vi "Q -- check range -- i -- real - window.vi"(4 "window":dbl=inf, 6 "center":dbl=-inf, 8 "default":dbl=nan, 11 "number":dbl=11.0) -> (0 "selector":T1, 2 "in range?":bool=TRUE, 3 "number in range":dbl)   [LabVIEW 2015]
uses:
  comparison control.ctl
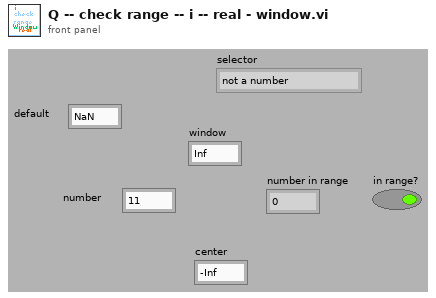
[diagram p1: front panel]
types:
  T1 = typedef "comparison control.ctl" = enum16{"not a number", "above", "in range", "below"}
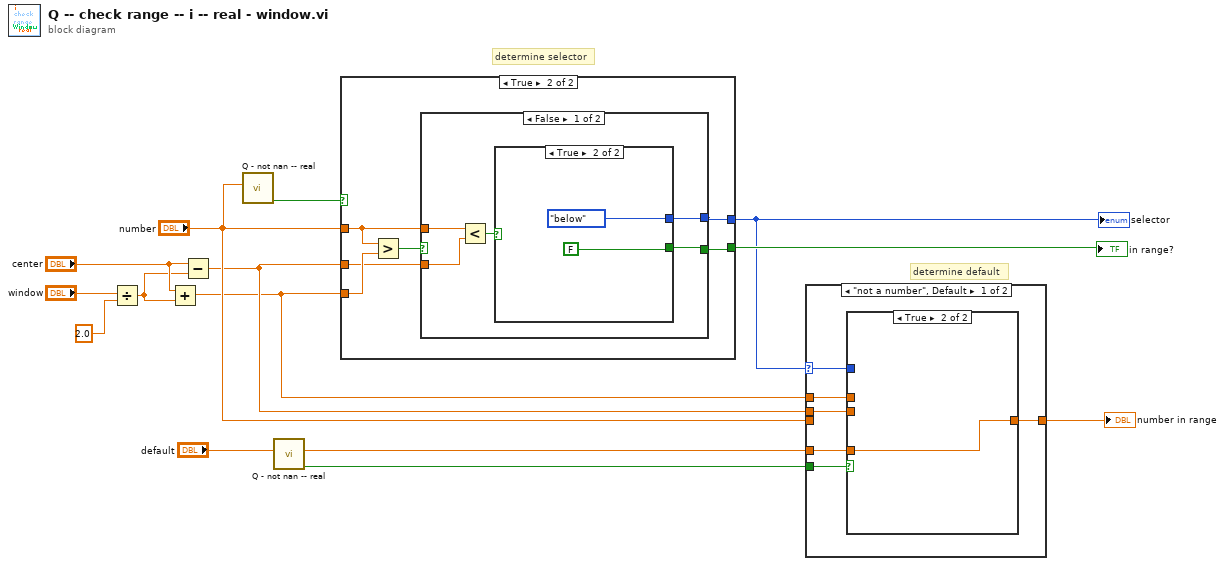
[diagram p0: block diagram]
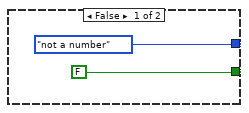
[diagram p5: hidden frame]
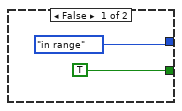
[diagram p6: hidden frame]
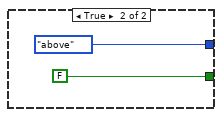
[diagram p7: hidden frame]
diagram:
  # "determine default"
  # "determine selector"
  n1 = Divide(x="window", y=2.0) -> (x/y=w3:dbl)
  n2 = Add(x="center", y=w3) -> (x+y=w1:dbl)
  n3 = Subtract(x="center", y=w3) -> (x-y=w2:dbl)
  n4 = call "Q - not nan -- real.vi"("Numeric"="number") -> ("Boolean"=w12:bool)  [unwired: 9 in, 1 out]
  n5 = call "Q - not nan -- real.vi"("Numeric"="default") -> ("Boolean"=w8:bool, "out"=w7:dbl)  [unwired: 9 in]
  n6 = case shown="True" w12 {
    tunnel: w1 -> [_ w21]
    tunnel: w2 -> [_ w18]
    tunnel: [FALSE w17] -> w14
    tunnel: [comparison_control."not a number" ("selector") w22] -> w11
    tunnel: "number" -> [_ w19]
    frame False {
    }
    frame True {
      n7 = Greater?(x=w19, y=w21) -> (0:w20:bool)
      n8 = case shown="False" w20 {
        tunnel: [w27 comparison_control."above" ("selector")] -> w22
        tunnel: w19 -> [w26 _]
        tunnel: w18 -> [w25 _]
        tunnel: [w23 FALSE] -> w17
        frame False {
          n9 = Less?(x=w26, y=w25) -> (x < y?=w24:bool)
          n10 = case shown="True" w24 {
            tunnel: [comparison_control."in range" ("selector") comparison_control."below" ("selector")] -> w27
            tunnel: [TRUE FALSE] -> w23
            frame False {
            }
            frame True {
            }
          }
        }
        frame True {
        }
      }
    }
  }
  "in range?" <- w14
  "selector" <- w11
  n11 = case shown="\"not a number\", Default" w11 {
    selector: w11 -> [w36 _]
    tunnel: [w38 w47] -> w10
    tunnel: "number" -> [_ w47]
    tunnel: w8 -> [w39 _]
    tunnel: w7 -> [w37 _]
    tunnel: w1 -> [w35 _]
    tunnel: w2 -> [w34 _]
    frame "not a number", Default {
      n12 = case shown="True" w39 {
        tunnel: [w42 w46] -> w38
        tunnel: w37 -> [_ w46]
        tunnel: w36 -> [w43 _]
        tunnel: w35 -> [w41 _]
        tunnel: w34 -> [w40 _]
        frame False {
          n13 = case shown="\"not a number\", Default" w43 {
            tunnel: [w44 w45] -> w42
            tunnel: w41 -> [_ w45]
            tunnel: w40 -> [w44 _]
            frame "not a number", Default {
            }
            frame "above" {
            }
          }
        }
        frame True {
        }
      }
    }
    frame "in range" {
    }
  }
  "number in range" <- w10
